vi "PwF_ToF_GetDataQuality.vi"(0 "PwF ToF Ref":T1, 11 "error in (no error)":errorcluster) -> (4 "PwF ToF Ref":T1, 6 "AmbLight":dbl, 10 "DistStdDev":dbl, 15 "error out":errorcluster)   [LabVIEW 2018]
uses:
  ToF_TypeDef/PwF ToF Ref.ctl
  ToF_TypeDef/PwF ToF RangingMode.ctl
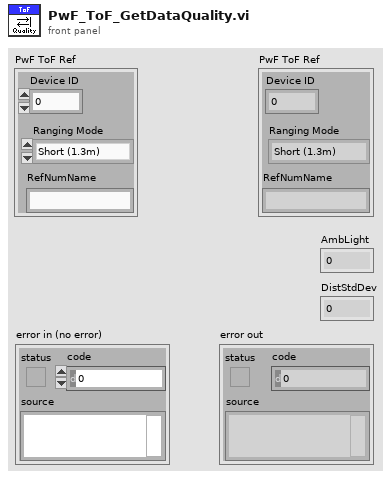
[diagram p1: front panel]
types:
  T1 = typedef "PwF ToF Ref.ctl" = cluster{"Device ID":u8, "Ranging Mode":T2, "RefNumName":string}
  T2 = typedef "PwF ToF RangingMode.ctl" = enum8{"Short (1.3m)", "Medium (2m)", "Long (4m)"}
  T3 = cluster{"Data[0]":u8, "Data[1]":u8, "Data[2]":u8, "Data[3]":u8, "Data[4]":u8, "Data[5]":u8, "Data[6]":u8, "Data[7]":u8, "Data[8]":u8}
  T4 = cluster{"Data[0]":u32, "Data[1]":u32, "Data[2]":u32, "Data[3]":u32, "Data[4]":u32, "Data[5]":u32, "Data[6]":u32, "Data[7]":u32, "Data[8]":u32}
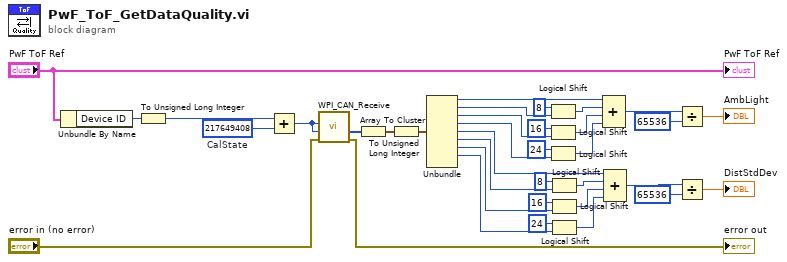
[diagram p0: block diagram]
diagram:
  w34 = u32 217649408  # CalState
  n1 = Unbundle By Name("PwF ToF Ref") -> ("Device ID"=w36:u8)
  n2 = To Unsigned Long Integer(number=w36) -> (unsigned 32bit integer=w29:u32)
  n3 = Add(x=w29, y=w34) -> (x+y=w33:u32)
  n4 = call <vilib>:"WPI_CAN_Receive.vi"("error in (no error)"="error in (no error)", "Message ID Mask"=w33, "Message ID"=w33) -> ("error out"=→"error out":errorcluster, "Data"=w32:u8[])  [unwired: 6 in, 1 out]
  n5 = Array To Cluster(array=w32) -> (cluster=w1:T3)
  n6 = To Unsigned Long Integer(number=w1) -> (unsigned 32bit integer=w18:T4)
  n7 = Unbundle(w18) -> ("Data[0]"=w24:u32, "Data[1]"=w25:u32, "Data[2]"=w22:u32, "Data[3]"=w21:u32, "Data[4]"=w11:u32, "Data[5]"=w10:u32, "Data[6]"=w9:u32, "Data[7]"=w8:u32)  [unwired: 1 out]
  n8 = Logical Shift(y=i16 8, x=w25) -> (x << y=w23:u32)
  n9 = Logical Shift(y=i16 16, x=w22) -> (x << y=w20:u32)
  n10 = Logical Shift(y=i16 24, x=w21) -> (x << y=w19:u32)
  n11 = Logical Shift(y=i16 8, x=w10) -> (x << y=w14:u32)
  n12 = Logical Shift(y=i16 16, x=w9) -> (x << y=w13:u32)
  n13 = Logical Shift(y=i16 24, x=w8) -> (x << y=w12:u32)
  n14 = Compound Arithmetic op=ADD(w24, w23, w20, w19) -> (w7:u32)
  n15 = Compound Arithmetic op=ADD(w11, w14, w13, w12) -> (w2:u32)
  n16 = Divide(x=w7, y=u32 65536) -> (x/y=→"AmbLight":dbl)
  n17 = Divide(x=w2, y=u32 65536) -> (x/y=→"DistStdDev":dbl)
  "PwF ToF Ref" <- "PwF ToF Ref"
